vi "多个线圈写入.vi"(8 "Error in":errorcluster caption="Error in (no error)", 9 "values":bool[](array[boolean]), 10 "starting address":u16, 11 "Slave ID":u8=10) -> (0 "error out":errorcluster)   [LabVIEW 2016, in "质控单元.lvlib"]
uses:
  <vilib>/Plasmionique/MB Master/MB_Master_Serial/MB_Master_Serial.lvclass
  F:/Program Files/National Instruments/LabVIEW 2016/vi.lib/Plasmionique/MB Master/MB_Master/MB_Master.lvclass
  <vilib>/Plasmionique/MB Master/MB Master.lvlib
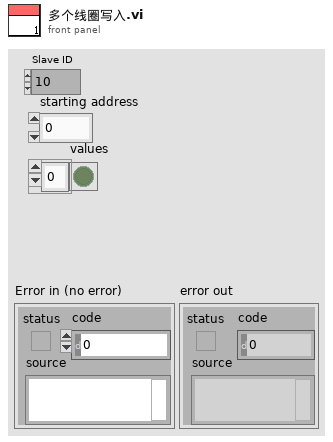
[diagram p1: front panel]
types:
  T1 = cluster{"baud rate (bps)":u32, "stop bits":u16, "parity":u16, "flow control":u16, "timeout":u32, "retries":i32}
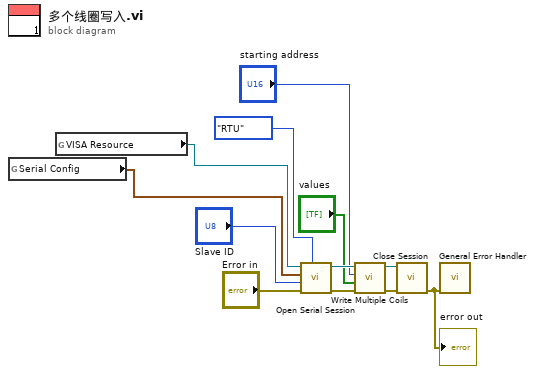
[diagram p0: block diagram]
diagram:
  n1 = global read "串口参数全局.vi" "Serial Config"() -> (w1:T1)
  n2 = global read "串口参数全局.vi" "VISA Resource"() -> (w2:refnum<visa-resource-name>)
  n3 = call <vilib>:"Open Serial Session.vi"("Mode (RTU)"=enum16{"RTU", "ASCII"}."RTU", "Error in"="Error in", "Slave ID"="Slave ID", "Serial Config"=w1, "VISA Resource"=w2) -> ("Error out"=w10:errorcluster, "MB_Serial session"=w9:refnum<class "MB_Master_Serial.lvclass">)  [unwired: 5 in]
  n4 = call <vilib>:"Write Multiple Coils.vi"("error in (no error)"=w10, "values"="values", "starting address"="starting address", "MB session in"=w9) -> ("error out"=w12:errorcluster, "MB session out"=w11:refnum<class "MB_Master_Serial.lvclass">)  [unwired: 6 in]
  n5 = call-dynamic "Close Session.vi"("error in (no error)"=w12, "MB_Serial session"=w11) -> ("error out"=w6:errorcluster)  [unwired: 9 in]
  "error out" <- w6
  n6 = call <vilib>:"General Error Handler.vi"("error in (no error)"=w6) -> ()  [unwired: 10 in, 5 out]
